vi "S2C_FORNAX_Proc_ReadMsg.vi"(8 "Error In":errorcluster) -> (0 "Error Out":errorcluster, 3 "Message":string)   [LabVIEW 2015]
doc: "Reads any TCP data from the Fornax communications connection."
uses:
  S2C_FORNAX_Proc_Globals.vi
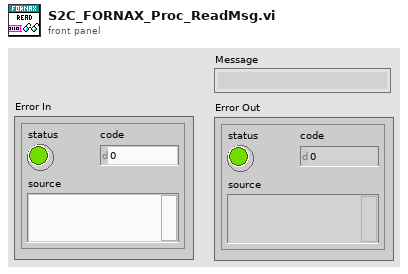
[diagram p1: front panel]
types:
  T1 = enum16{"Standard", "Buffered", "CRLF", "Immediate"}
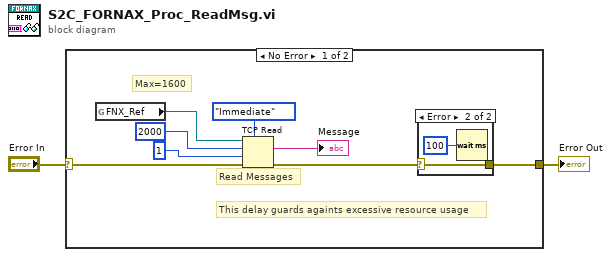
[diagram p0: block diagram]
diagram:
  n1 = case shown="No Error" "Error In" {
    selector: "Error In" -> [w7 w14]
    tunnel: [w5 w14] -> w1
    frame No Error {
      # "Max=1600"
      # "This delay guards againts excessive resource usage"
      # "Read Messages"
      n2 = global read "S2C_FORNAX_Proc_Globals.vi" "FNX_Ref"() -> (w8:refnum<k5>)
      n3 = TCP Read(connection ID=w8, bytes to read=2000, error in (no error)=w7, 7:T1."Immediate" ("mode (standard)"), 9:1 ("timeout ms (25000)")) -> (data out=→"Message":string, error out=w6:errorcluster)  [unwired: 1 out]
      n4 = case shown="Error" w6 {
        selector: w6 -> [w11 w13]
        tunnel: [w11 w13] -> w5
        frame No Error {
        }
        frame Error {
          n5 = Wait (ms)(milliseconds to wait=u32 100) -> ()  [unwired: 1 out]
        }
      }
    }
    frame Error {
    }
  }
  "Error Out" <- w1
